vi "HGF_SVSubscriber.AppendData2Variant.vi"(0 "initData":variant, 1 "shared variable refnum":refnum<k21>, 2 "typeDescriptor":string, 3 "typeOfSVService (monitored)":T1=4 items=["ONCE_ONLY"=1, "TIMED"=2, "MONITORED"=4], 4 "timeout [0s]":i32, 5 "error in (no error)":errorcluster, 7 "stamped (T)":bool=TRUE) -> (14 "dup initData":variant, 19 "error out":errorcluster)   [LabVIEW 2012, in "HGF_SV.lvlib" / "HGF_SVSubscriber.lvclass"]
uses:
  HGF_SVSubscriber.lvclass
  DimLVEvent/LVDimInterface/LVDimInterface.dim service type.ctl
  DimLVEvent/LVDimInterface/LVDimInterface.lvlib
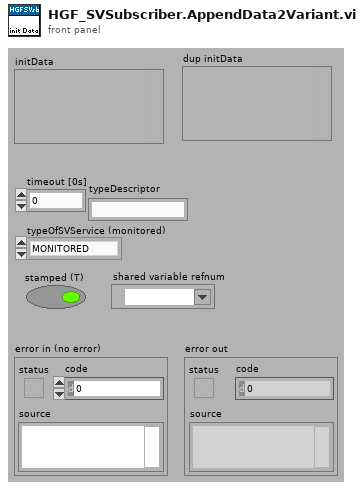
[diagram p1: front panel]
types:
  T1 = typedef "LVDimInterface.lvlib/LVDimInterface.dim service type.ctl" = u16
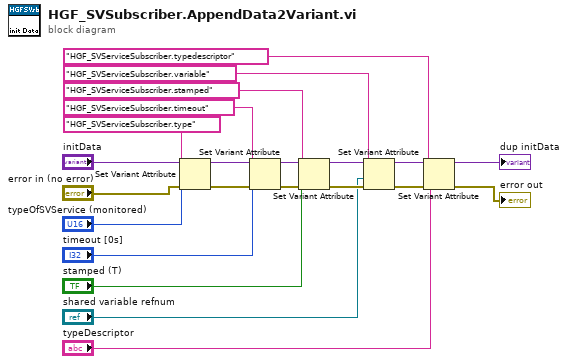
[diagram p0: block diagram]
diagram:
  n1 = Set Variant Attribute(Variant="initData", name="HGF_SVServiceSubscriber.type", value="typeOfSVService (monitored)", error in="error in (no error)") -> (Variant out=w15:variant, error out=w17:errorcluster)  [unwired: 1 out]
  n2 = Set Variant Attribute(Variant=w15, name="HGF_SVServiceSubscriber.timeout", value="timeout [0s]", error in=w17) -> (Variant out=w16:variant, error out=w18:errorcluster)  [unwired: 1 out]
  n3 = Set Variant Attribute(Variant=w16, name="HGF_SVServiceSubscriber.stamped", value="stamped (T)", error in=w18) -> (Variant out=w10:variant, error out=w9:errorcluster)  [unwired: 1 out]
  n4 = Set Variant Attribute(Variant=w10, name="HGF_SVServiceSubscriber.variable", value="shared variable refnum", error in=w9) -> (Variant out=w3:variant, error out=w2:errorcluster)  [unwired: 1 out]
  n5 = Set Variant Attribute(Variant=w3, name="HGF_SVServiceSubscriber.typedescriptor", value="typeDescriptor", error in=w2) -> (Variant out=→"dup initData":variant, error out=→"error out":errorcluster)  [unwired: 1 out]
